vi "Run.vi"(8 "error in (no error)":errorcluster caption="entrée d'erreur (pas d'erreur)", 10 "Image":u16(ring) items=["China", "Flower"], 11 "Load_SampleImage en entrée":refnum<class "Load_SampleImage.lvclass">) -> (0 "error out":errorcluster caption="sortie d'erreur", 3 "Load_SampleImage en entrée":refnum<class "Load_SampleImage.lvclass">)   [LabVIEW 2020, in "Load_SampleImage.lvclass"]
doc: "Scikit-learn intègre également quelques exemples d'images JPEG publiées sous licence Creative Commons par leurs auteurs. Ces images peuvent être utiles pour tester des algorithmes et un pipeline sur des données 2D.\n\nWarning : The default coding of images is based on the uint8 dtype to spare memory. Often machine learning algorithms work best if the input is converted to a floating point representation first. Also, if you plan to use matplotlib.pyplpt.imshow don’t forget to scale to the range 0 - 1 as done in the following example.\n\nReturns :\n\n- images : list of ndarray of shape (427, 640, 3)\nThe two sample image china and flower."
uses:
  Load_SampleImage.lvclass
  Load_SampleImage.lvclass/Load_SampleImage.ctl
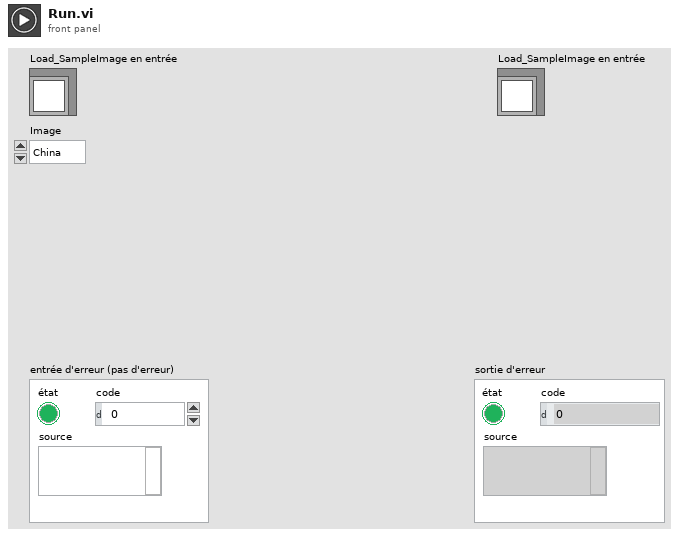
[diagram p1: front panel]
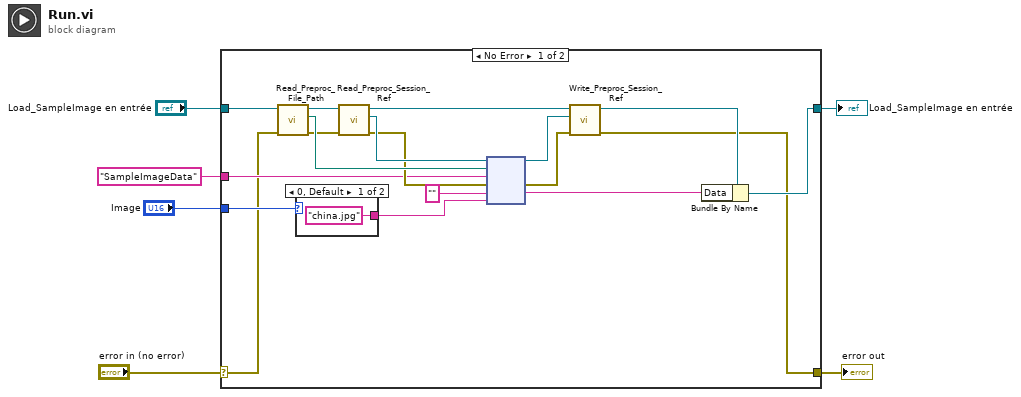
[diagram p0: block diagram]
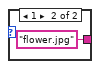
[diagram p2: hidden frame]
diagram:
  n1 = case shown="No Error" "error in (no error)" {
    selector: "error in (no error)" -> [w10 w28]
    tunnel: [w7 w28] -> w5
    tunnel: [w8 w27] -> w3
    tunnel: "Load_SampleImage en entrée" -> [w13 w27]
    tunnel: "SampleImageData" -> [w12 _]
    tunnel: "Image" -> [w11 _]
    frame No Error {
      n2 = call-dynamic "Read_Preproc_File_Path.vi"("error in (no error)"=w10, "Python in"=w13) -> ("error out"=w19:errorcluster, "File_Path"=w22:path, "Python out"=w24:refnum<class "Load_SampleImage.lvclass">)  [unwired: 7 in]
      n3 = case shown="0, Default" w11 {
        tunnel: ["china.jpg" "flower.jpg"] -> w15
        frame 0, Default {
        }
        frame 1 {
        }
      }
      n4 = call-dynamic "Read_Preproc_Session_Ref.vi"("error in (no error)"=w19, "Python in"=w24) -> ("error out"=w20:errorcluster, "Session_ref"=w21:refnum<k35>, "Python out"=w23:refnum<class "Load_SampleImage.lvclass">)  [unwired: 7 in]
      n5 = node(w21, w22, w12, w20, "", w15) -> (w16:refnum<k35>, w18:errorcluster, w9:string)  [unwired: 1 in, 2 out]
      n6 = call-dynamic "Write_Preproc_Session_Ref.vi"("error in (no error)"=w18, "Session_ref"=w16, "Python in"=w23) -> ("error out"=w7:errorcluster, "Python out"=w14:refnum<class "Load_SampleImage.lvclass">)  [unwired: 7 in]
      n7 = Bundle By Name(cluster=w14, "Data"=w9) -> (w8:refnum<class "Load_SampleImage.lvclass">)
    }
    frame Error {
    }
  }
  "error out" <- w5
  "Load_SampleImage en entrée" <- w3
